vi "Multiplexer_Ch_No.vi"(0 "Channel Number":i16) -> (1 "Multiplexer Ch No":i16, 2 "ADC Ch No":i16)   [LabVIEW 2012]
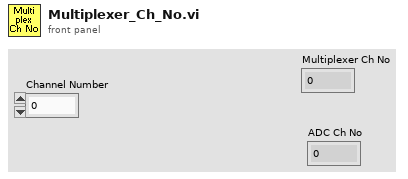
[diagram p1: front panel]
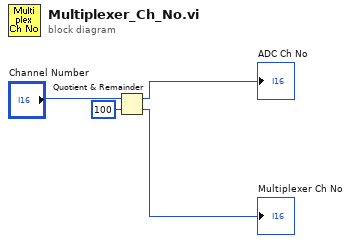
[diagram p0: block diagram]
diagram:
  n1 = Quotient & Remainder(x="Channel Number", y=i16 100) -> (x-y*floor(x/y)=→"ADC Ch No":i16, floor(x/y)=→"Multiplexer Ch No":i16)
